vi "Feature_Scorer(CuLab).vi"(4 "Feature Scorer Params":T27={"Nearest_Neihbours"=1, "Calculate Anomaly Map"=TRUE, "Gaussian_Blur"={"Kernel_Size"=33, "sigma"=4.0}}, 8 "error in":errorcluster, 9 "bs, h, w, c1+..cN":i32[](array[numeric]), 10 "embedding":refnum<class "T2D_SGL.lvclass">, 11 "PCore_Instance":T1 {"NN out"."LR_Update_Policy"."WarmUp_Ratio" min=1; "NN out"."LR_Update_Policy"."WarmUp_Iter" min=1; "NN out"."LR_Update_Policy"."LR0" format="%.7f"; "Dataset_Stats"."vars"."R" format="%#_3g"; "Dataset_Stats"."vars"."G" format="%#_3g"; "Dataset_Stats"."vars"."B" format="%#_3g"; "Dataset_Stats"."means"."R" format="%#_3g"; "Dataset_Stats"."means"."G" format="%#_3g"; "Dataset_Stats"."means"."B" format="%#_3g"}) -> (0 "error out":errorcluster, 1 "anomaly map":refnum<class "T3D_SGL.lvclass">, 2 "pred score":refnum<class "T1D_SGL.lvclass">, 3 "PCore_Instance out":T1 {"NN out"."LR_Update_Policy"."WarmUp_Ratio" min=1; "NN out"."LR_Update_Policy"."WarmUp_Iter" min=1; "NN out"."LR_Update_Policy"."LR0" format="%.7f"; "Dataset_Stats"."vars"."R" format="%#_3g"; "Dataset_Stats"."vars"."G" format="%#_3g"; "Dataset_Stats"."vars"."B" format="%#_3g"; "Dataset_Stats"."means"."R" format="%#_3g"; "Dataset_Stats"."means"."G" format="%#_3g"; "Dataset_Stats"."means"."B" format="%#_3g"}, 5 "dT(pCore)":dbl)   [LabVIEW 2020]
uses:
  API/Controls/Feature_Scorer_Params.ctl
  API/Controls/Gaussian_Blur.ctl
  <vilib>/Ngene/CuLab - GPU Accelerated Toolkit/Toolkit/Low_Level/Tensor_Classes/T_Children/T2D/T2D_Children/T2D_SGL/T2D_SGL.lvclass
  C:/Program Files/National Instruments/LabVIEW 2020/vi.lib/Ngene/CuLab - GPU Accelerated Toolkit/Toolkit/Low_Level/Tensor_Classes/T_Children/T2D/T2D.lvclass
  <vilib>/Ngene/CuLab - GPU Accelerated Toolkit/Toolkit/Low_Level/Tensor_Classes/T_Children/T1D/T1D_Children/T1D_SGL/T1D_SGL.lvclass
  API/Controls/PatchCore_Instance.ctl
  API/Controls/PatchCore_DS_Stats.ctl
  API/Controls/Image_Stats_RGB.ctl
  <vilib>/Ngene/Deep Learning Toolkit/Toolkit/NN_Network/Controls/NN.ctl
  <vilib>/Ngene/Deep Learning Toolkit/Toolkit/NN_Layers/Controls/NN_Layer_ref.ctl
  <vilib>/Ngene/Deep Learning Toolkit/Toolkit/NN_Layers/Controls/NN_Layer.ctl
  <vilib>/Ngene/Deep Learning Toolkit/Toolkit/NN_Layers/Controls/NN_Layer_Type.ctl
  <vilib>/Ngene/Deep Learning Toolkit/Toolkit/NN_Data/API/NN_Dims(C,H,W).ctl
  <vilib>/Ngene/Deep Learning Toolkit/Toolkit/NN_Layers/Controls/NN_Layer_Metrics.ctl
  <vilib>/Ngene/Deep Learning Toolkit/Toolkit/NN_Network/Controls/NN_Device.ctl
  <vilib>/Ngene/Deep Learning Toolkit/Toolkit/NNg/cuda/Controls/nng_cuda_handles.ctl
  <vilib>/Ngene/Deep Learning Toolkit/Toolkit/NN_Layers/Controls/NN_Layer_Dimty.ctl
  <vilib>/Ngene/Deep Learning Toolkit/Toolkit/NN_Layers/Controls/NN_Layer_RF_State.ctl
  <vilib>/Ngene/Deep Learning Toolkit/Toolkit/NN_Data/API/NN_Dims(V,H).ctl
  <vilib>/Ngene/Deep Learning Toolkit/Toolkit/NN_Network/Controls/NN_In_Out_Dim-ty.ctl
  <vilib>/Ngene/Deep Learning Toolkit/Toolkit/NN_Train/Controls/NN_Train_Params.ctl
  <vilib>/Ngene/Deep Learning Toolkit/Toolkit/NN_Train/Controls/NN_Train_Optimizer.ctl
  <vilib>/Ngene/Deep Learning Toolkit/Toolkit/NN_Train/Controls/NN_Train_Data_Sampling.ctl
  <vilib>/Ngene/Deep Learning Toolkit/Toolkit/NN_Train/Controls/NN_LR_Policy_Cfg.ctl
  <vilib>/Ngene/Deep Learning Toolkit/Toolkit/NN_Train/Controls/NN_LR_Policy_Type.ctl
  <vilib>/Ngene/Deep Learning Toolkit/Toolkit/NN_Train/Controls/NN_Train_Session_Data.ctl
  <vilib>/Ngene/Deep Learning Toolkit/Toolkit/NN_Data/Controls/NN_Ground_truth.ctl
  <vilib>/Ngene/Deep Learning Toolkit/Toolkit/NN_Train/Controls/NN_Loss_Type.ctl
  <vilib>/Ngene/Deep Learning Toolkit/Toolkit/NNg/Network/WS/Controls/NNG_WS.ctl
  <vilib>/Ngene/Deep Learning Toolkit/Toolkit/NNg/Network/WS/Controls/NNg_WS_Mem_DVR.ctl
  <vilib>/Ngene/Deep Learning Toolkit/Toolkit/NNg/cuda/Controls/cuda_Mem_desc.ctl
  API/Controls/PCore_Device.ctl
  API/Controls/PatchCore_Init_CFG.ctl
  API/Controls/PatchCore_BackBone_Selector.ctl
  API/Controls/Coreset_Params.ctl
  API/Controls/Random_Projection_Coreset.ctl
  API/Controls/MemBank_and_Norm_Variants.ctl
  <vilib>/Ngene/CuLab - GPU Accelerated Toolkit/Toolkit/Low_Level/Tensor_Classes/T_Children/T3D/T3D_Children/T3D_SGL/T3D_SGL.lvclass
  <vilib>/Ngene/CuLab - GPU Accelerated Toolkit/Toolkit/Low_Level/Tensor_Classes/T_Children/T3D/Controls/T3D_Dims.ctl
  <vilib>/Utility/High Resolution Relative Seconds.vi
  Euclidean_Dist_with_MemBank(CuLab).vi
  <vilib>/Ngene/CuLab - GPU Accelerated Toolkit/Toolkit/API/Array/CU_Array_Size.vi
  <vilib>/Ngene/CuLab - GPU Accelerated Toolkit/Toolkit/API/Array/Array Size/CU_Array_Size_T2D.vi
  <vilib>/Ngene/CuLab - GPU Accelerated Toolkit/Toolkit/API/Array/Reshape Array  (API)/CU_Reshape_to_T1D.vi
  <vilib>/Ngene/CuLab - GPU Accelerated Toolkit/Toolkit/API/Array/Reshape Array  (API)/CU_Reshape_to_T1D/T2D/CU_Reshape_to_T1D_(T2D_SGL).vi
  <vilib>/Ngene/CuLab - GPU Accelerated Toolkit/Toolkit/API/Signal Processing/Signal Operation/CU_Decimate_Single_Shot_Adaptive.vi
  <vilib>/Ngene/CuLab - GPU Accelerated Toolkit/Toolkit/API/Signal Processing/Signal Operation/Decimate (single shot) adaptive/CU_Decimate_Single_Shot_Adaptive_T1D_SGL.vi
  <vilib>/Ngene/CuLab - GPU Accelerated Toolkit/Toolkit/API/Array/Reshape Array  (API)/CU_Reshape_to_T3D/T1D/CU_Reshape_to_T3D_(T1D_SGL).vi
  <vilib>/Ngene/CuLab - GPU Accelerated Toolkit/Toolkit/CuLab.lvlib
  <vilib>/Ngene/Deep Learning Toolkit/Toolkit/Deep_Learning_Toolkit_by_Ngene.lvlib
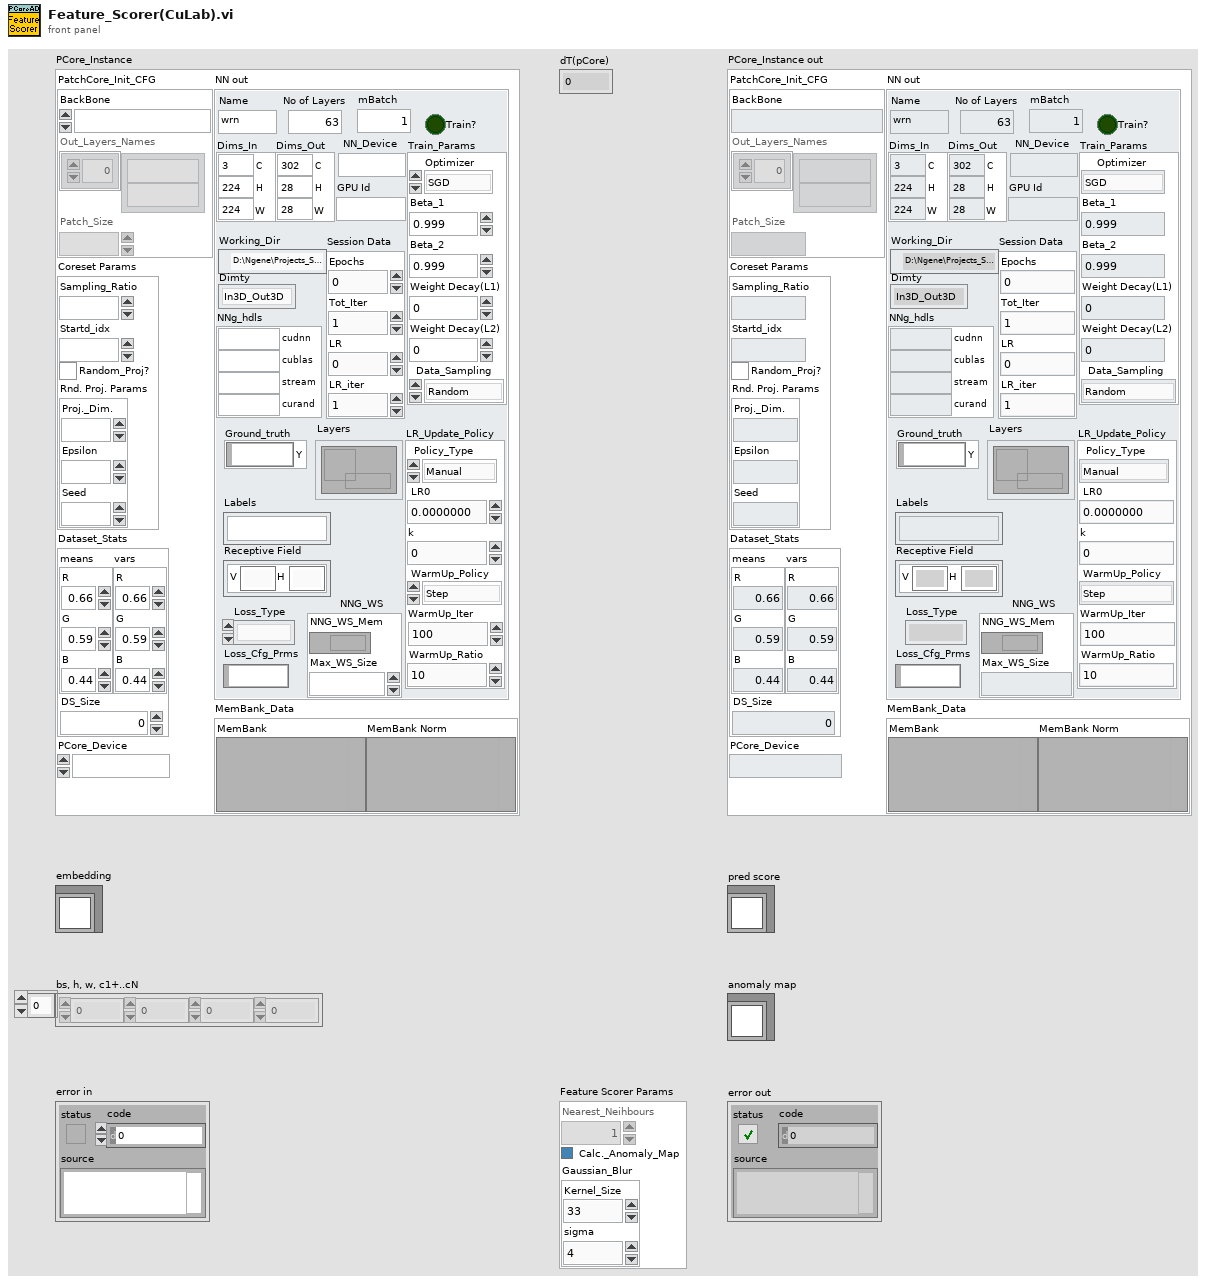
[diagram p1: front panel]
types:
  T1 = typedef "PatchCore_Instance.ctl" = cluster{"Dataset_Stats":T2, "NN":T4, "PCore_Device":T21, "PatchCore_Init_CFG":T22, "Coreset Params":T24, "MemBank_Data":T26}
  T2 = typedef "PatchCore_DS_Stats.ctl" = cluster{"means":T3, "vars":T3, "DS_Size":i32}
  T3 = typedef "Image_Stats_RGB.ctl" = cluster{"R":sgl, "G":sgl, "B":sgl}
  T4 = typedef "Deep_Learning_Toolkit_by_Ngene.lvlib/NN.ctl" = cluster{"Name":string, "No of Layers":i32, "mBatch":i32, "Layers":T5[], "Dimty":T6, "Dims_In":T7, "Dims_Out":T7, "Working_Dir":path, "Train?":bool, "Train_Params":T8, "LR_Update_Policy":T11, "Session Data":T13, "Ground_truth":T14, "NNg_hdls":T15, "NN_Device":T16, "GPU Id":i32, "Labels":string[], "Receptive Field":T17[], "Loss_Type":T18, "Loss_Cfg_Prms":variant, "NNG_WS":T19}
  T5 = typedef "Deep_Learning_Toolkit_by_Ngene.lvlib/NN_Layer_ref.ctl" = refnum<data-value>
  T6 = typedef "Deep_Learning_Toolkit_by_Ngene.lvlib/NN_In_Out_Dim-ty.ctl" = enum8{"In1D_Out1D", "In3D_Out1D", "In3D_Out3D", "In3D_OutBBox"}
  T7 = typedef "Deep_Learning_Toolkit_by_Ngene.lvlib/NN_Dims(C,H,W).ctl" = cluster{"C":i32, "H":i32, "W":i32}
  T8 = typedef "Deep_Learning_Toolkit_by_Ngene.lvlib/NN_Train_Params.ctl" = cluster{"Optimizer":T9, "Beta_1":sgl, "Beta_2":sgl, "Weight Decay(L1)":sgl, "Weight Decay(L2)":sgl, "Data_Sampling":T10}
  T9 = typedef "Deep_Learning_Toolkit_by_Ngene.lvlib/NN_Train_Optimizer.ctl" = enum16{"SGD", "Adam", "Adagrad", "Adadelta", "RMSProp", "Nesterov"}
  T10 = typedef "Deep_Learning_Toolkit_by_Ngene.lvlib/NN_Train_Data_Sampling.ctl" = enum16{"Random", "Sequential"}
  T11 = typedef "Deep_Learning_Toolkit_by_Ngene.lvlib/NN_LR_Policy_Cfg.ctl" = cluster{"Policy_Type":T12, "LR0":dbl, "k":sgl, "WarmUp_Policy":enum16{"Step", "Ramp"}, "WarmUp_Iter":i32, "WarmUp_Ratio":sgl}
  T12 = typedef "Deep_Learning_Toolkit_by_Ngene.lvlib/NN_LR_Policy_Type.ctl" = enum16{"Manual", "Step", "Exp", "1/t"}
  T13 = typedef "Deep_Learning_Toolkit_by_Ngene.lvlib/NN_Train_Session_Data.ctl" = cluster{"Epochs":sgl, "Tot_Iter":i32, "LR":sgl, "LR_iter":i32}
  T14 = typedef "Deep_Learning_Toolkit_by_Ngene.lvlib/NN_Ground_truth.ctl" = cluster{"Y":variant}
  T15 = typedef "Deep_Learning_Toolkit_by_Ngene.lvlib/nng_cuda_handles.ctl" = cluster{"cudnn":u64, "cublas":u64, "stream":u64, "curand":u64}
  T16 = typedef "Deep_Learning_Toolkit_by_Ngene.lvlib/NN_Device.ctl" = enum16{"CPU", "GPU"}
  T17 = typedef "Deep_Learning_Toolkit_by_Ngene.lvlib/NN_Dims(V,H).ctl" = cluster{"V":i32, "H":i32}
  T18 = typedef "Deep_Learning_Toolkit_by_Ngene.lvlib/NN_Loss_Type.ctl" = enum16{"None", "MSE", "CrossEntropy", "YOLO_v2", "YOLO_v4"}
  T19 = typedef "Deep_Learning_Toolkit_by_Ngene.lvlib/NNG_WS.ctl" = cluster{"NNG_WS_Mem":T20, "Max_WS_Size":i64}
  T20 = typedef "Deep_Learning_Toolkit_by_Ngene.lvlib/NNg_WS_Mem_DVR.ctl" = refnum<data-value>
  T21 = typedef "PCore_Device.ctl" = enum16{"CPU", "GPU(CuLab)"}
  T22 = typedef "PatchCore_Init_CFG.ctl" = cluster{"BackBone":T23, "Out_Layers_Names":string[], "Patch_Size":u32}
  T23 = typedef "PatchCore_BackBone_Selector.ctl" = enum16{"WRN_50_2_L2L3"}
  T24 = typedef "Coreset_Params.ctl" = cluster{"Sampling_Ratio":sgl, "Startd_idx":i32, "Random_Proj?":bool, "Rnd. Proj. Params":T25}
  T25 = typedef "Random_Projection_Coreset.ctl" = cluster{"Proj._Dim.":i32, "Epsilon":sgl, "Seed":i32}
  T26 = typedef "MemBank_and_Norm_Variants.ctl" = cluster{"MemBank":variant, "MemBank Norm":variant}
  T27 = typedef "Feature_Scorer_Params.ctl" = cluster{"Nearest_Neihbours":i32, "Calculate Anomaly Map":bool, "Gaussian_Blur":T28}
  T28 = typedef "Gaussian_Blur.ctl" = cluster{"Kernel_Size":i32, "sigma":sgl}
  T29 = typedef "CuLab.lvlib/T3D_Dims.ctl" = cluster{"C ":i32, "H":i32, "W":i32}
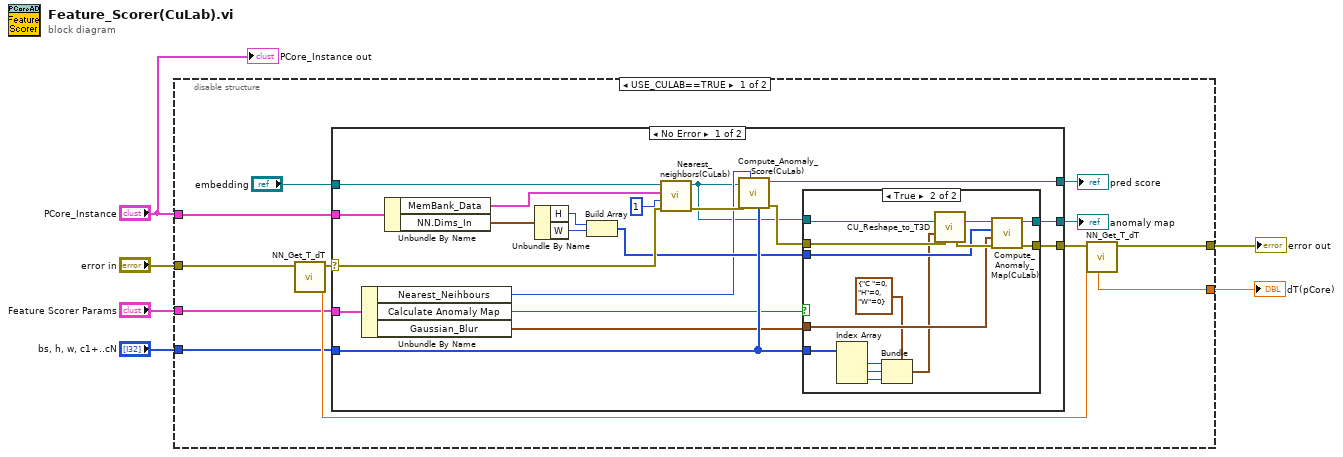
[diagram p0: block diagram]
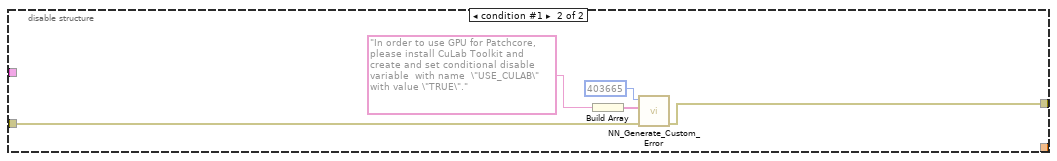
[diagram p4: hidden frame]
diagram:
  n1 = disable-structure shown="USE_CULAB==TRUE" {
    disable-tunnel: "error in" -> [w12 w56]
    disable-tunnel: "Feature Scorer Params" -> [w11 _]
    disable-tunnel: "bs, h, w, c1+..cN" -> [w10 _]
    disable-tunnel: "PCore_Instance" -> [w9 _]
    disable-tunnel: [w8 w55] -> w2
    disable-tunnel: [w7 _] -> w1
    frame condition #0 (active) {
      n2 = call <vilib>:"NN_Get_T_dT.vi"("error in (no error)"=w12) -> ("T_out"=w13:dbl, "error out"=w14:errorcluster)  [unwired: 6 in, 1 out]
      n3 = case shown="No Error" w14 {
        selector: w14 -> [w36 w54]
        tunnel: w10 -> [w33 _]
        tunnel: [w20 _] -> w17
        tunnel: [w31 _] -> w15
        tunnel: [w29 w54] -> w18
        tunnel: "embedding" -> [w35 _]
        tunnel: w11 -> [w27 _]
        tunnel: w9 -> [w23 _]
        frame No Error {
          n4 = Unbundle By Name(w27) -> ("Nearest_Neihbours"=w26:i32, "Calculate Anomaly Map"=w25:bool, "Gaussian_Blur"=w24:T28)
          n5 = Unbundle By Name(w23) -> ("MemBank_Data"=w22:T26, "NN.Dims_In"=w21:T7)
          n6 = Unbundle By Name(w21) -> ("H"=w38:i32, "W"=w37:i32)
          n7 = Build Array(w38, w37) -> (w32:i32[])
          n8 = call "Nearest_neighbors(CuLab).vi"("error in"=w36, "n neighbors"=1, "Membank"=w22, "Features"=w35) -> ("error out"=w34:errorcluster, "patch scores"=w19:refnum<class "T1D_SGL.lvclass">)  [unwired: 5 in, 1 out]
          n9 = call "Compute_Anomaly_Score(CuLab).vi"("bs, h, w, c1+..cN"=w33, "n neighbors"=w26, "error in"=w34, "patch scores"=w19) -> ("error out"=w30:errorcluster, "image-lvl anomaly score"=w20:refnum<class "T1D_SGL.lvclass">)  [unwired: 6 in]
          n10 = case shown="True" w25 {
            tunnel: [_ w43] -> w31
            tunnel: [w39 w42] -> w29
            tunnel: w24 -> [_ w45]
            tunnel: w32 -> [_ w46]
            tunnel: w19 -> [_ w51]
            tunnel: w33 -> [_ w53]
            tunnel: w30 -> [w39 w48]
            frame False {
            }
            frame True {
              n11 = Index Array(array=w53) -> (element #1=w52:i32, element #2=w50:i32, element #3=w49:i32)  [unwired: 3 in]
              n12 = Bundle(cluster=T29 {"C "=0, "H"=0, "W"=0} ("Dest Dims"), "C"=w52, "H"=w50, "W"=w49) -> (w41:T29)
              n13 = call-poly <vilib>:"CU_Reshape_to_T3D.vi"("Tensor in"=w51, "Dest Dims"=w41, "error in (no error)"=w48) -> ("Dest out"=w44:refnum<class "T3D_SGL.lvclass">, "error out"=w47:errorcluster)  [unwired: 11 in]
              n14 = call "Compute_Anomaly_Map(CuLab).vi"("error in"=w47, "Gaussian Blur"=w45, "input img size"=w46, "patch scores [bs,w,h]"=w44) -> ("error out"=w42:errorcluster, "anomaly map"=w43:refnum<class "T3D_SGL.lvclass">)  [unwired: 6 in]
            }
          }
        }
        frame Error {
        }
      }
      "pred score" <- w17
      "anomaly map" <- w15
      n15 = call <vilib>:"NN_Get_T_dT.vi"("T_in"=w13, "error in (no error)"=w18) -> ("error out"=w8:errorcluster, "dT"=w7:dbl)  [unwired: 5 in, 1 out]
    }
    frame condition #1 {
      n16 = Build Array("In order to use GPU for Patchcore, please install CuLab Toolkit and create and set conditional disable variable  with name  \"USE_CULAB\" with value \"TRUE\"." ("Message")) -> (w58:string[])
      n17 = call <vilib>:"NN_Generate_Custom_Error.vi"("error in (no error)"=w56, "Message"=w58, "Error_code"=403665) -> ("error out"=w55:errorcluster)  [unwired: 8 in]
    }
  }
  "error out" <- w2
  "dT(pCore)" <- w1
  "PCore_Instance out" <- "PCore_Instance"
